vi "Pack For Grpc.vi"(8 "error in (no error)":errorcluster, 9 "Configuration / Resuls (Config)":enum16{"Configuration", "Results"}(ring), 10 "Data Value":variant, 11 "Measurement Customizations in":refnum<class "MeasurementPlugin.lvclass">) -> (0 "error out":errorcluster, 2 "Any":T1, 3 "Measurement Customizations out":refnum<class "MeasurementPlugin.lvclass">)   [LabVIEW 2021, in "Single Tone Measurements_Class D Amplifier.lvlib" / "MeasurementPlugin.lvclass"]
uses:
  MeasurementPlugin.lvclass
  <vilib>/gRPC/LabVIEW gRPC Library/Shared/Any.ctl
  Measurement Configuration.ctl
  shared/controls/digital audio protocol/data justification.ctl
  shared/controls/digital audio protocol/endianness.ctl
  shared/controls/digital audio protocol/digital edge.ctl
  shared/controls/digital audio protocol/logic level.ctl
  shared/controls/output mode.ctl
  shared/controls/weighting filter.ctl
  shared/controls/lowpass filter.ctl
  shared/controls/highpass filter.ctl
  Measurement Results.ctl
  2eca732d-dbaa-43bf-a7dd-ede2da65bc1b.vi
  a6012965-5700-4384-8228-972e71b6560c.vi
  <vilib>/gRPC/LabVIEW gRPC Library/Server API/Translate Protobuf Error.vi
  <vilib>/AdvancedString/1D String Array to Delimited String.vi
  <vilib>/gRPC/LabVIEW gRPC Library/Server API/Server/Get Server DLL Path.vi
  Single Tone Measurements_Class D Amplifier.lvlib
  <vilib>/gRPC/LabVIEW gRPC Library/grpc-lvsupport-release.lvlib
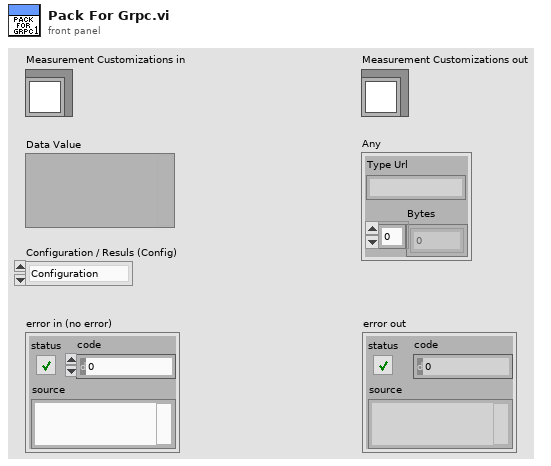
[diagram p1: front panel]
types:
  T1 = typedef "grpc-lvsupport-release.lvlib/Any.ctl" = cluster{"Type Url":string, "Bytes":u8[]}
  T2 = typedef "grpc-lvsupport-release.lvlib/grpcId.ctl" = u64
  T3 = typedef "Single Tone Measurements_Class D Amplifier.lvlib/Measurement Configuration.ctl" = cluster{"digital channel list":string, "frame clock rate":dbl, "number of channels":u32, "channel length":u32, "bit depth":u32, "data justification":T4, "endianness":T5, "bit clock edge sync":T6, "frame sync edge for channel 0":T6, "channel 0 offset":u32, "master clock channel list":string, "master clock rate":dbl, "logic level":T7, "signal frequency":dbl, "output mode":T8, "output level (dB)":dbl, "output power (W)":dbl, "output range (pk-pk)":dbl, "load impedance":dbl, "signal phase":dbl, "acq sampling rate":dbl, "min measurement cycles":u32, "min measurement time (s)":dbl, "min settling cycles":u32, "min settling time (s)":dbl, "acq channel":string, "band start":dbl, "band stop":dbl, "weighting filter":T9, "lowpass filter":T10, "highpass filter":T11}
  T4 = typedef "data justification.ctl" = enum32{"Left Justified", "Right Justified"}
  T5 = typedef "endianness.ctl" = enum32{"MSB First", "LSB First"}
  T6 = typedef "digital edge.ctl" = enum32{"Rising", "Falling"}
  T7 = typedef "logic level.ctl" = enum32{"3.3 V", "1.8 V", "1.2 V"}
  T8 = typedef "output mode.ctl" = enum32{"Level", "Power"}
  T9 = typedef "weighting filter.ctl" = enum32{"Linear", "A-weighting", "B-weighting", "C-weighting"}
  T10 = typedef "lowpass filter.ctl" = enum32{"No filter", "AES17 20kHz", "AES17 40kHz"}
  T11 = typedef "highpass filter.ctl" = enum32{"DC", "AC"}
  T12 = typedef "Single Tone Measurements_Class D Amplifier.lvlib/Measurement Results.ctl" = cluster{"Channel name":string, "Calculated frequency (Hz)":dbl, "Calculated amplitude (dB)":dbl, "SNR (dB)":dbl, "THD+N (dB)":dbl, "THD (dB)":dbl, "Dynamic range (dB)":dbl, "Gain error (dB)":dbl, "SFDR (dB)":dbl, "Output power (W)":dbl, "wfm - t0":dbl, "wfm - dt":dbl, "wfm - data":dbl[], "fft - f0":dbl, "fft - df":dbl, "fft - data":dbl[]}
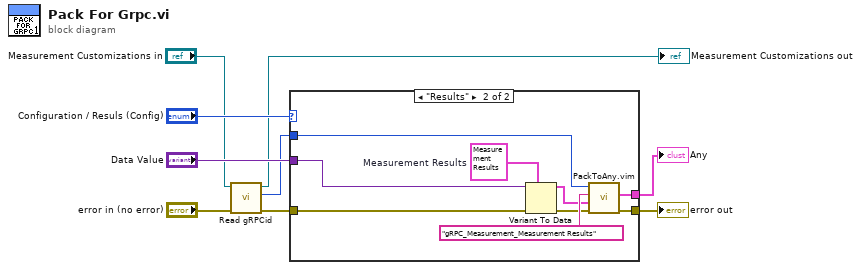
[diagram p0: block diagram]
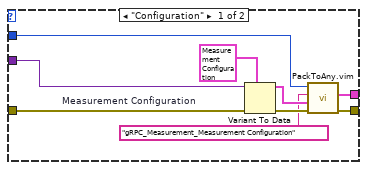
[diagram p2: hidden frame]
diagram:
  n1 = call-dynamic "Read gRPCid.vi"("error in (no error)"="error in (no error)", "MeasurementPluginService in"="Measurement Customizations in") -> ("error out"=w4:errorcluster, "gRPCid"=w1:T2, "MeasurementPluginService out"=→"Measurement Customizations out":refnum<class "MeasurementPlugin.lvclass">)  [unwired: 7 in]
  n2 = case shown="\"Results\"" "Configuration / Resuls (Config)" {
    tunnel: w4 -> [w18 w27]
    tunnel: "Data Value" -> [w17 w26]
    tunnel: w1 -> [w14 w22]
    tunnel: [w16 w24] -> w8
    tunnel: [w15 w23] -> w7
    frame "Configuration" {
      w11 = T3 {"digital channel list"="7821\\PCMo 8", "frame clock rate"=48000.0, "number of channels"=2, "channel length"=32, "bit depth"=24, "data justification"=enum."Left Justified", "endianness"=enum."MSB First", "bit clock edge sync"=enum."Rising", "frame sync edge for channel 0"=enum."Rising", "channel 0 offset"=1, "master clock channel list"="7821\\PCMo 0", "master clock rate"=12288000.0, "logic level"=enum."3.3 V", "signal frequency"=1000.0, "output mode"=enum."Level", "output level (dB)"=4.0, "output power (W)"=1.0, "output range (pk-pk)"=3.16, "load impedance"=4.0, "signal phase"=0.0, "acq sampling rate"=1000.0, "min measurement cycles"=1000, "min measurement time (s)"=5.0, "min settling cycles"=0, "min settling time (s)"=0.0, "acq channel"="", "band start"=20.0, "band stop"=20000.0, "weighting filter"=enum."Linear", "lowpass filter"=enum."No filter", "highpass filter"=enum."DC"}  # Measurement Configuration
      n3 = Variant To Data(error in=w18, type=w11, Variant=w17) -> (data=w13:T3, error out=w12:errorcluster)
      n4 = call "PackToAny.vim"("error in"=w12, "Data To Pack"=w13, "Message Type"="gRPC_Measurement_Measurement Configuration", "gRPCid in"=w14) -> ("error out"=w16:errorcluster, "Any"=w15:T1)  [unwired: 5 in, 1 out]
    }
    frame "Results" {
      w25 = T12 {"Channel name"="", "Calculated frequency (Hz)"=0.0, "Calculated amplitude (dB)"=0.0, "SNR (dB)"=0.0, "THD+N (dB)"=0.0, "THD (dB)"=0.0, "Dynamic range (dB)"=0.0, "Gain error (dB)"=0.0, "SFDR (dB)"=0.0, "Output power (W)"=0.0, "wfm - t0"=0.0, "wfm - dt"=0.0, "wfm - data"=[], "fft - f0"=0.0, "fft - df"=0.0, "fft - data"=[]}  # Measurement Results
      n5 = Variant To Data(error in=w27, type=w25, Variant=w26) -> (data=w20:T12, error out=w19:errorcluster)
      n6 = call "PackToAny.vim"("error in"=w19, "Data To Pack"=w20, "Message Type"="gRPC_Measurement_Measurement Results", "gRPCid in"=w22) -> ("error out"=w24:errorcluster, "Any"=w23:T1)  [unwired: 5 in, 1 out]
    }
  }
  "error out" <- w8
  "Any" <- w7
